vi "uA_daq_Test_uA_Vol_Loging_testing.vi"() -> ()   [LabVIEW 2015]
uses:
  <vilib>/DAQmx/read.llb/DAQmx Read.vi
  <vilib>/DAQmx/read.llb/DAQmx Read (Analog 1D Wfm NChan NSamp).vi
  <vilib>/DAQmx/miscellaneous.llb/DAQmx Fill In Error Info.vi
panel:
  out "Vbat":dbl
  out "uA Current":dbl
  out "VBat_ext":waveform(dbl)(graph)
  in  "USB DAQ":tag
  out "Task out":refnum<k21>="Stop"
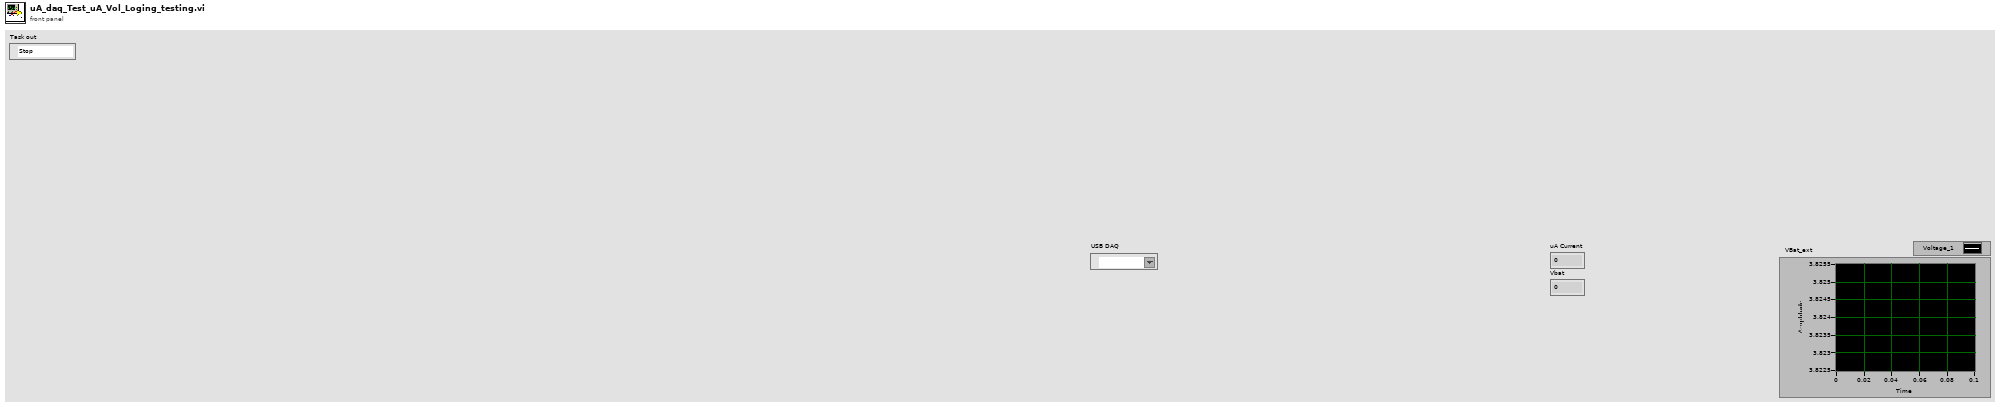
[diagram p1: front panel]
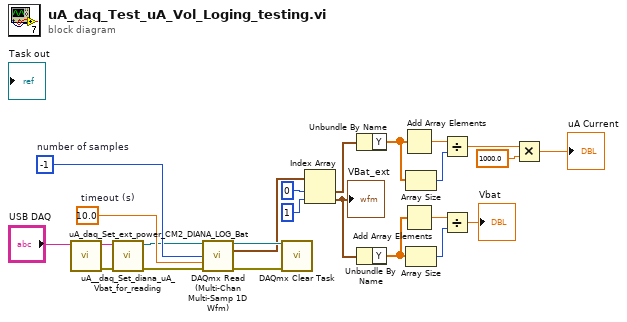
[diagram p0: block diagram]
diagram:
  w23 = 10.0  # timeout (s)
  w24 = -1  # number of samples
  n1 = call "uA_daq_Set_ext_power_CM2_DIANA_LOG_Bat.vi"("USB DAQ in"="USB DAQ") -> ("error out"=w15:errorcluster, "USB DAQ out"=w7:tag)  [unwired: 9 in]
  n2 = call "uA__daq_Set_diana_uA_Vbat_for_reading.vi"("error in (no error)"=w15, "USB DAQ in"=w7) -> ("error out"=w19:errorcluster, "Refnum out"=w20:refnum<k21>)  [unwired: 8 in]
  n3 = call-poly "DAQmx Read (Multi-Chan Multi-Samp 1D Wfm).vi"("task/channels in"=w20, "number of samples per channel"=w24, "timeout"=w23, "error in"=w19) -> ("task out"=w21:refnum<k21>, "data"=w18:waveform(dbl)[], "error out"=w22:errorcluster)  [unwired: 9 in]
  n4 = call <vilib>:"DAQmx Clear Task.vi"("task in"=w21, "error in"=w22) -> ()  [unwired: 13 in, 1 out]
  n5 = Index Array(array=w18, index #1=0 ("index"), index #2=1 ("index")) -> (element #1=w14:waveform(dbl), element #2=w3:waveform(dbl))
  "VBat_ext" <- w3
  n6 = Unbundle By Name(w14) -> ("Y"=w12:dbl[])
  n7 = Unbundle By Name(w3) -> ("Y"=w5:dbl[])
  n8 = Add Array Elements(numeric array=w12) -> (sum=w13:dbl)
  n9 = Add Array Elements(numeric array=w5) -> (sum=w4:dbl)
  n10 = Array Size(array=w12) -> (size(s)=w11:i32)
  n11 = Array Size(array=w5) -> (size(s)=w6:i32)
  n12 = Divide(x=w13, y=w11) -> (x/y=w10:dbl)
  n13 = Divide(x=w4, y=w6) -> (x/y=→"Vbat":dbl)
  n14 = Multiply(x=w10, y=1000.0) -> (x*y=→"uA Current":dbl)
